vi "CALC_MARK_DIST.vi"(0 "VISA IN":refnum<visa-resource-name>, 1 "Markey number":i32, 2 "Marker Distance":i32, 5 "error in":errorcluster, 7 "Channel":i32) -> (14 "VISA Out":refnum<visa-resource-name>, 19 "error out":errorcluster)   [LabVIEW 2018, in "PNA-X.lvlib"]
doc: "CALCulate<cnum>:MARKer<mkr>:DISTance <num> \n(Read-Write) Set or query marker distance on a time domain trace. \nThe Write command moves the marker to the specified distance value. Once moved, you can read the \nY axis value or read the X-axis time value. (Distance is calculated from the X-axis time value.) \nThe Read command reads the distance of the marker. \nIf the marker is set as delta, the WRITE and READ data is relative to the reference marker. \nSee Critical Note \nParameters \n<cnum> Channel number of the measurement. There must be a selected measurement \non that channel. If unspecified, <cnum> is set to 1. \n<mkr> Any existing marker number from 1 to 10; if unspecified, value is set to 1. \n<num> Marker distance in the unit of measure specified with \nCALC:TRAN:TIME:MARK:UNIT \nExamples CALC:MARK:DIST .1 \ncalculate2:marker8:distance 5 \nQuery Syntax CALCulate<cnum>:MARKer<mkr>:DISTance? \nReturn Type Numeric \nDefault Not Applicable"
uses:
  PNA-X.lvlib
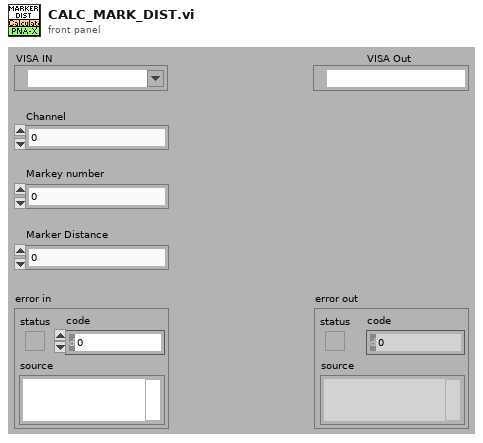
[diagram p1: front panel]
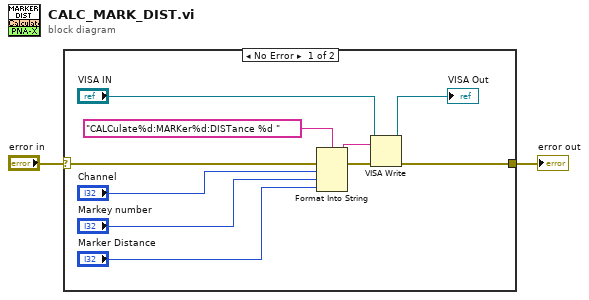
[diagram p0: block diagram]
diagram:
  n1 = case shown="No Error" "error in" {
    selector: "error in" -> [w12 w13]
    tunnel: [w7 w13] -> w1
    frame No Error {
      n2 = Format Into String(format string="CALCulate%d:MARKer%d:DISTance %d " ("Cmdline"), error in=w12, "Channel", "Markey number", "Marker Distance") -> (resulting string=w10:string, error out=w11:errorcluster)  [unwired: 1 in]
      n3 = VISA Write(VISA resource name="VISA IN", write buffer=w10, error in (no error)=w11) -> (VISA resource name out=→"VISA Out":refnum<visa-resource-name>, error out=w7:errorcluster)  [unwired: 1 out]
    }
    frame Error {
    }
  }
  "error out" <- w1
